vi "DFD Non-Uniform Filter Bank Decomposition (Array).vi"(7 "init? (F)":bool, 8 "error in (no error)":errorcluster, 10 "filter bank in":T1 {"mFBank_SynthesisFilters"."mMRate_SumWl" min=1 max=32 step=1; "mFBank_SynthesisFilters"."mMRate_InputIwl" min=1 max=32 step=1; "mFBank_SynthesisFilters"."mMRate_GainWl" min=1 max=32 step=1; "mFBank_SynthesisFilters"."mMRate_OutputWl" min=1 max=32 step=1; "mFBank_SynthesisFilters"."mMRate_InputWl" min=1 max=32 step=1; "mFBank_SynthesisFilters"."mMRate_CoefWl" min=1 max=32 step=1; "mFBank_SynthesisFilters"."mMRate_Mode" items=["Default"=-1, "No Rate Change"=0, "Interpolation"=1, "Decimation"=2, "Interpolated"=3, "Rational"=4]; "mFBank_AnalysisFilters"."mMRate_SumWl" min=1 max=32 step=1; "mFBank_AnalysisFilters"."mMRate_InputIwl" min=1 max=32 step=1; "mFBank_AnalysisFilters"."mMRate_GainWl" min=1 max=32 step=1; "mFBank_AnalysisFilters"."mMRate_OutputWl" min=1 max=32 step=1; "mFBank_AnalysisFilters"."mMRate_InputWl" min=1 max=32 step=1; "mFBank_AnalysisFilters"."mMRate_CoefWl" min=1 max=32 step=1; "mFBank_AnalysisFilters"."mMRate_Mode" items=["Default"=-1, "No Rate Change"=0, "Interpolation"=1, "Decimation"=2, "Interpolated"=3, "Rational"=4]; "mFBank_Type" items=["Uniform", "Non-Uniform"]}, 11 "x":dbl[](array[numeric]) format="%.2f") -> (0 "error out":errorcluster, 3 "M bands":cluster{"band":dbl[]}[](array[cluster]))   [LabVIEW 2023]
doc: "Filters the input sequence <B>x</B> using an M-band analysis bank specified by <B>analysis bank</B> continuously. The initial internal states are controlled by <B>init? (F)</B>.\n\nYou can call the VIs in <B>Filter Bank Design</B> sub-palette to design a filter bank."
uses:
  <vilib>/addons/Digital Filter Design/FilterBank.llb/Object/DFD Filter Bank Obj.ctl
  <vilib>/addons/Digital Filter Design/_Objects.llb/DFD Multirate Filter Obj.ctl
  <vilib>/addons/Digital Filter Design/_Objects.llb/DFD Multirate Mode.ctl
  <vilib>/addons/Digital Filter Design/_Objects.llb/DFD Coef Norm Type.ctl
  <vilib>/addons/Digital Filter Design/_Objects.llb/DFD Round-off Mode.ctl
  <vilib>/addons/Digital Filter Design/_Objects.llb/DFD FXP MRate Multiply Mode.ctl
  <vilib>/addons/Digital Filter Design/FilterBank.llb/Object/DFD Filter Bank Processing Method.ctl
  <vilib>/addons/Digital Filter Design/FilterBank.llb/Object/DFD Filter Bank Type.ctl
  <vilib>/addons/Digital Filter Design/Multirate.llb/DFD MRate Filtering with State (Array).vi
  <vilib>/addons/Digital Filter Design/NI_DigFilterLicensed.lvlib
  <vilib>/addons/Digital Filter Design/NI_DigFilter_FilterBank.lvlib
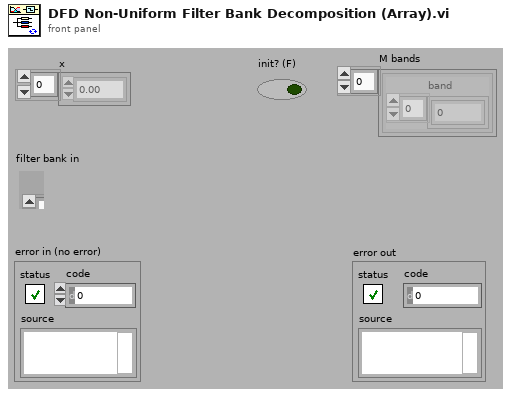
[diagram p1: front panel]
types:
  T1 = typedef "NI_DigFilter_FilterBank.lvlib/DFD Filter Bank Obj.ctl" = cluster{"mFBank_AnalysisFilters":T2[], "mFBank_SynthesisFilters":T2[], "mFBank_#Bands":i32, "mFBank_ProcMethod":T7, "mFBank_Coeffs":dbl[], "mFBank_Gain":dbl, "mFBank_Delay":i32, "mFBank_Type":T8}
  T2 = typedef "NI_DigFilterLicensed.lvlib/DFD Multirate Filter Obj.ctl" = cluster{"mMRate_Structure":enum16{"CIC", "FIR", "IIR", "Lattice"}, "mMRate_Mode":T3, "mMRate_Factor":i32, "mMRate_FIRParams":cluster{"mMRate_FIR_H":dbl[], "mMRate_FIR_IsNyquist?":bool, "mMRate_FIR_IsSymmetric?":bool}, "mMRate_CICParams":cluster{"mMRate_CIC_#Stage":i32, "mMRate_CIC_Lag":i32, "mMRate_CIC_Type":enum16{"Lowpass", "Highpass"}}, "mMRate_Order":i32, "mMRate_Version":string, "mMRate_Comments":string, "mMRate_RationalFactor":cluster{"mMRate_L":i32, "mMRate_M":i32}, "mMRate_Fs":dbl, "mMRate_Quantized?":bool, "mMRate_QFilterGain":dbl, "mMRate_CoefWl":i16, "mMRate_Scaling":cluster{"mMRate_ScaleByPowerOf2?":bool, "mMRate_ScaleType":T4}, "mMRate_InputWl":i16, "mMRate_OutputWl":i16, "mMRate_OutputMode":T5, "mMRate_MultMode":T6, "mMRate_BitPruning":bool, "mMRate_GainWl":i16, "mMRate_OutputFwl":i16, "mMRate_SumIwl":i16, "mMRate_InputIwl ":i16, "mMRate_SumWl":i16, "mMRate_CoefIwl":i16}
  T3 = typedef "NI_DigFilterLicensed.lvlib/DFD Multirate Mode.ctl" = i16
  T4 = typedef "NI_DigFilterLicensed.lvlib/DFD Coef Norm Type.ctl" = enum16{"No Norm", "Time Domain 1-Norm", "Time Domain 2-Norm", "Time Domain Inf-Norm"}
  T5 = typedef "NI_DigFilterLicensed.lvlib/DFD Round-off Mode.ctl" = enum16{"Nearest", "Truncation"}
  T6 = typedef "NI_DigFilterLicensed.lvlib/DFD FXP MRate Multiply Mode.ctl" = enum16{"Truncated", "Full"}
  T7 = typedef "NI_DigFilter_FilterBank.lvlib/DFD Filter Bank Processing Method.ctl" = enum16{"General", "2-Band QMF Lattice", "Cosine-Modulated"}
  T8 = typedef "NI_DigFilter_FilterBank.lvlib/DFD Filter Bank Type.ctl" = u16
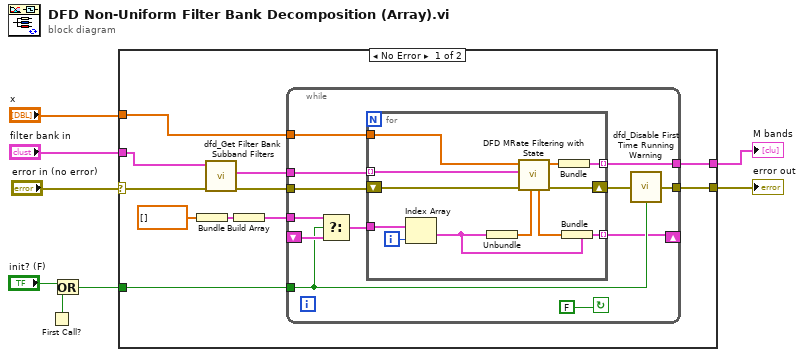
[diagram p0: block diagram]
diagram:
  n1 = First Call?() -> (First Call?: T/F=w4:bool)
  n2 = Or(x="init? (F)", y=w4) -> (x .or. y?=w2:bool)
  n3 = case shown="No Error" "error in (no error)" {
    selector: "error in (no error)" -> [w12 w44]
    tunnel: "filter bank in" -> [w13 _]
    tunnel: "x" -> [w16 _]
    tunnel: [w15 w44] -> w5
    tunnel: w2 -> [w14 _]
    tunnel: [w9 _] -> w1
    frame No Error {
      n4 = Bundle(dbl[] []) -> (w18:cluster{dbl[]})  [unwired: 1 in]
      n5 = call <vilib>:"dfd_Get Filter Bank Subband Filters.vi"("error in (no error)"=w12, "filter bank in"=w13) -> ("error out"=w11:errorcluster, "analysis filters"=w10:T2[])  [unwired: 6 in, 2 out]
      n6 = Build Array(w18) -> (w17:cluster{dbl[]}[])
      n7 = while {
        tunnel: w10 -> [w23]
        tunnel: w11 -> [w24]
        shift-right: [w25] -> _
        shift-left: _ -> [w30]
        tunnel: w14 -> [w27]
        tunnel: w17 -> [w31]
        tunnel: w16 -> [w22]
        tunnel: [w28] -> w15
        tunnel: [w21] -> w9
        stop <- FALSE continue-if-true
        n8 = Select(t=w31, s=w27, f=w30) -> (s? t:f=w26:cluster{dbl[]}[])
        n9 = for {
          tunnel: w22 -> [w43]
          tunnel: w23 -> [w38] mode=indexing
          shift-right: [w42] -> w20
          shift-left: w24 -> [w39]
          tunnel: [w32] -> w21 mode=indexing
          tunnel: w26 -> [w36]
          tunnel: [w33] -> w25 mode=indexing
          i -> [w35]
          n10 = Index Array(array=w36, index=w35) -> (element=w34:cluster{dbl[]})
          n11 = Unbundle(w34) -> (w37:dbl[])
          n12 = call-poly <vilib>:"DFD MRate Filtering with State.vi"("state in"=w37, "error in (no error)"=w39, "multirate filter"=w38, "signal in"=w43) -> ("error out"=w42:errorcluster, "signal out"=w40:dbl[], "state out"=w41:dbl[])  [unwired: 5 in]
          n13 = Bundle("signal out"=w40) -> (w32:cluster{"signal out":dbl[]})  [unwired: 1 in]
          n14 = Bundle(cluster=w34, w41) -> (w33:cluster{dbl[]})
        }
        n15 = call <vilib>:"dfd_Disable First Time Running Warning.vi"("error in"=w20, "disable?"=w27) -> ("error out"=w28:errorcluster)
      }
    }
    frame Error {
    }
  }
  "error out" <- w5
  "M bands" <- w1
